vi "CSGaussmeter.setUnit.vi"(0 "i ref in":refnum<vi>, 7 "Unit":T1, 11 "error in (no error)":errorcluster) -> (4 "i ref out":refnum<vi>, 15 "error out":errorcluster)   [LabVIEW 2014, in "CSGaussmeter.lvlib"]
doc: "This VI sets the Unit off T, G, A/m.\n\n\nDurch das VI kann die Einheit gewechselt werden (T, G, A/m)."
uses:
  CSGaussmeter.lvlib
  instr.lib/FH_55/TypeDef/Unit.ctl
  CS_Core/CSObj/CSObj.lvlib
  CSlibraries/UtilityLib/UtilityLib.lvlib
  instr.lib/FH_55/FH 55.lvlib
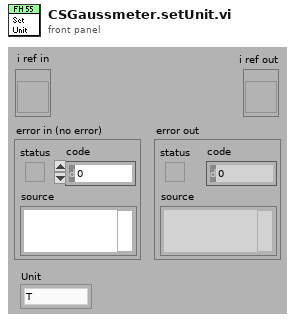
[diagram p1: front panel]
types:
  T1 = typedef "FH 55.lvlib/Unit.ctl" = enum16{"T", "G", "A/m"}
  T2 = typedef "CSGaussmeter.lvlib/CSGaussmeter.i attribute.ctl" = cluster{"Name":string, "VISA Resource Name":refnum<visa-resource-name>, "actValues":cluster{" Limit":bool, "Unit ":T1, "Temp_Unit":T3, "Max":T4, " Filter":bool, " Peak":bool, " Auto_Range":bool, "Range":T5, " Rel":bool, " CTemp":bool, " CField":bool, "AC_DC ":bool, "Set_lower":cluster{"Numeric":dbl, "Cancel Button":bool, "Unit":T6}, "Set_upper":cluster{"Numeric":dbl, "Cancel Button":bool, "Unit":T6}, "Set_Rel":cluster{"Numeric":dbl, "Cancel Button":bool, "Unit":T6}, "Zero":bool, " Local":bool, "Reset":bool, " Init":bool}, "FH 55 Gauss-/Teslameter":T7, "MAX_Value":T8, "MIN_Value":T8, "Rel_Value":T8, "Array ":string[], "LIMU":dbl, " LIML":dbl, "Messwerte 2":string, "Messwerte ":cluster{"Numeric":i32, "OK Button":bool}, "serviceID":cluster{"Current ID":i32, "Unit ID":i32, "Temp ID":i32, "Name ID \n":i32, "Visa ID ":i32}, "setValues ":cluster{" Limit":bool, "Unit ":T1, "Temp_Unit":T3, "Max":T4, " Filter":bool, " Peak":bool, " Auto_Range":bool, "Range":T5, " Rel":bool, " CTemp":bool, " CField":bool, "AC_DC ":bool, "Set_lower":cluster{"Numeric":dbl, "Cancel Button":bool, "Unit":T6}, "Set_upper":cluster{"Numeric":dbl, "Cancel Button":bool, "Unit":T6}, "Set_Rel":cluster{"Numeric":dbl, "Cancel Button":bool, "Unit":T6}, "Zero":bool, " Local":bool, "Reset":bool, " Init":bool}}
  T3 = typedef "FH 55.lvlib/Temp_Unit.ctl" = enum16{"Temp off", "Celsius", "Fahrenheit"}
  T4 = typedef "FH 55.lvlib/Max.ctl" = enum16{"MAX off", "Show MAX", "MAX/MIN"}
  T5 = typedef "FH 55.lvlib/Range.ctl" = enum16{"1", "2", "3", "4", "5", "6", "7"}
  T6 = typedef "FH 55.lvlib/Unit2.ctl" = enum16{"mT", "G", "kA/m"}
  T7 = typedef "FH 55.lvlib/Display.ctl" = cluster{"current value":string, "Limit":string, "Remote":string, "function ":string, "Cluster":cluster{"AC/DC":string, "Auto":string, "Filter":string, "Range":string, "Rel":string, "Peak":string}}
  T8 = typedef "FH 55.lvlib/Value_String.ctl" = cluster{"Numeric":dbl, "String":string}
  T9 = cluster{"VISA Resource Name":refnum<visa-resource-name>}
  T10 = typedef "FH 55.lvlib/VisaCluster.ctl" = cluster{"VISA Resource Name":refnum<visa-resource-name>}
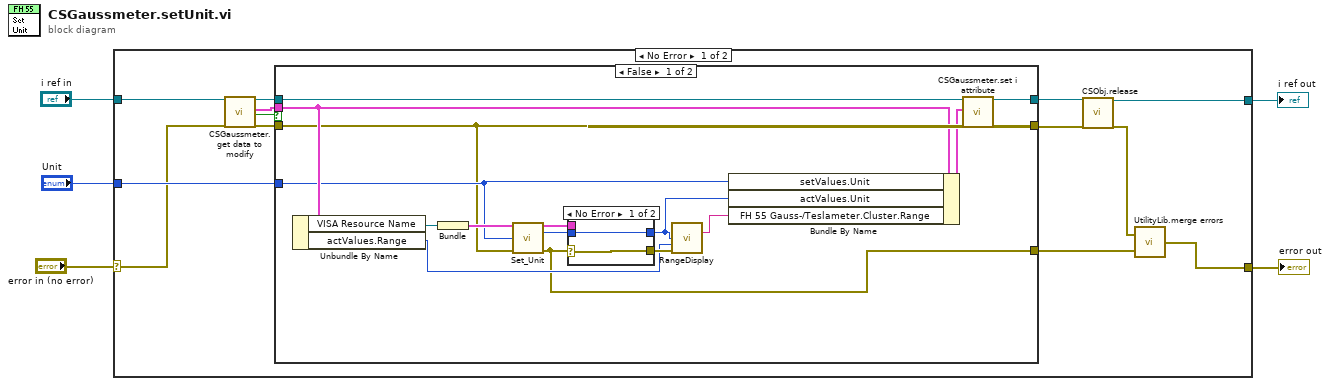
[diagram p0: block diagram]
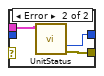
[diagram p2: hidden frame]
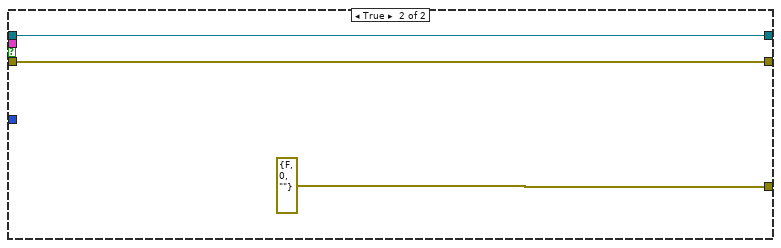
[diagram p3: hidden frame]
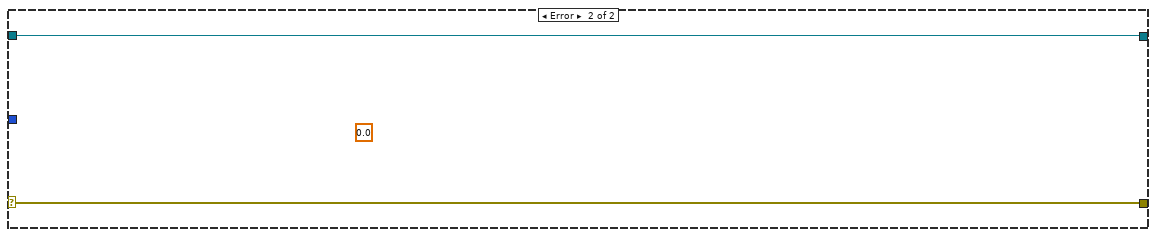
[diagram p4: hidden frame]
diagram:
  n1 = case shown="No Error" "error in (no error)" {
    selector: "error in (no error)" -> [w12 w43]
    tunnel: [w13 w43] -> w1
    tunnel: "i ref in" -> [w11 w44]
    tunnel: [w6 w44] -> w2
    tunnel: "Unit" -> [w15 _]
    frame No Error {
      n2 = call "CSGaussmeter.get data to modify.vi"("i ref in"=w11, "error in (no error)"=w12) -> ("i ref out"=w10:refnum<vi>, "i attribute"=w9:T2, "timed out"=w8:bool, "error out"=w7:errorcluster)  [unwired: 14 in]
      n3 = case shown="False" w8 {
        tunnel: w10 -> [w30 w41]
        tunnel: w7 -> [w26 w42]
        tunnel: w9 -> [w33 _]
        tunnel: [w25 w42] -> w16
        tunnel: [w28 w41] -> w18
        tunnel: w15 -> [w31 _]
        tunnel: [w20 errorcluster {"status"=FALSE, "code"=0, "source"=""} ("error out")] -> w14
        frame False {
          n4 = Unbundle By Name(w33) -> ("VISA Resource Name"=w34:refnum<visa-resource-name>, "actValues.Range"=w21:T5)
          n5 = Bundle("VISA Resource Name"=w34) -> (w32:T9)  [unwired: 1 in]
          n6 = call "Set_Unit.vi"("VisaCluster"=w32, "Unit"=w31, "error in (no error)"=w26) -> ("VisaCluster"=w22:T10, "Unit"=w24:T1, "error out"=w20:errorcluster)  [unwired: 9 in, 1 out]
          n7 = case shown="No Error" w20 {
            selector: w20 -> [w35 _]
            tunnel: w24 -> [w36 _]
            tunnel: [w36 w38] -> w19
            tunnel: [w35 w39] -> w23
            tunnel: w22 -> [_ w37]
            frame No Error {
            }
            frame Error {
              n8 = call "UnitStatus.vi"("VisaCluster"=w37) -> ("Unit"=w38:T1, "error out"=w39:errorcluster)  [unwired: 11 in, 2 out]
            }
          }
          n9 = call "RangeDisplay.vi"("Unit"=w19, "Range"=w21, "error in (no error)"=w23) -> ("Display"=w27:string)  [unwired: 10 in, 2 out]
          n10 = Bundle By Name(cluster=w33, "setValues.Unit"=w31, "actValues.Unit"=w19, "FH 55 Gauss-/Teslameter.Cluster.Range"=w27) -> (w29:T2)
          n11 = call "CSGaussmeter.set i attribute.vi"("i ref in"=w30, "i attribute"=w29, "error in (no error)"=w26) -> ("i ref out"=w28:refnum<vi>, "error out"=w25:errorcluster)  [unwired: 15 in]
        }
        frame True {
        }
      }
      n12 = call "CSObj.release.vi"("i ref in"=w18, "error in (no error)"=w16) -> ("i ref out"=w6:refnum<vi>, "error out"=w17:errorcluster)  [unwired: 16 in]
      n13 = call "UtilityLib.merge errors.vi"("error2 (no error)"=w14, "error1 (no error)"=w17) -> ("error out"=w13:errorcluster)
    }
    frame Error {
      (unwired) 0.0 ("Mid Setting [A or T]")
    }
  }
  "i ref out" <- w2
  "error out" <- w1
